vi "Configure Chan Group.vi"(8 "error in (no error)":errorcluster, 11 "Cfg Grandmaster in":refnum<class "Cfg Grandmaster.lvclass">) -> (0 "error out":errorcluster, 3 "Cfg Grandmaster out":refnum<class "Cfg Grandmaster.lvclass">)   [LabVIEW 2018, in "Configuration Grandmaster.lvlib" / "Cfg Grandmaster.lvclass"]
uses:
  Cfg Grandmaster.lvclass
  Cfg Grandmaster.lvclass/Cfg Grandmaster.ctl
  Class Chassis BOM/Chassis BOM.lvclass/Chassis BOM.ctl
  Class Chassis BOM/Read Chassis Alias.vi
  Class Chassis Cfg/ChassisCfg.lvclass
  Class Chassis BOM/Chassis BOM.lvclass
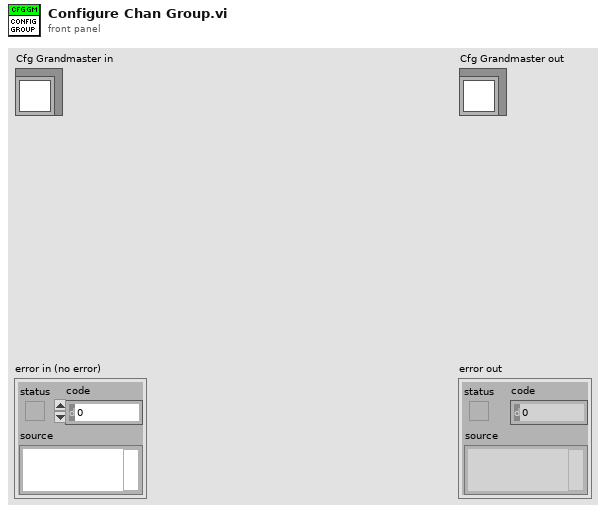
[diagram p1: front panel]
types:
  T1 = typedef "DAQMan Mode.ctl" = enum16{"Cfg", "Run", "Shutting Down"}
  T2 = typedef "ge_Cfg wChassis.ctl" = cluster{"Chassis BOM":refnum<class "Chassis BOM.lvclass">, "Chassis Cfg":refnum<class "ChassisCfg.lvclass">, "Chassis Tasks":refnum<class "Chassis Tasks.lvclass">, "HW Error":bool, "Unsvd Chgs?":bool}
  T3 = typedef "Selected Group.ctl" = cluster{"ChanGroup":i32, "Rate Class":T4}
  T4 = typedef "TE_Designator.ctl" = enum16{"High Speed", "Low Speed"}
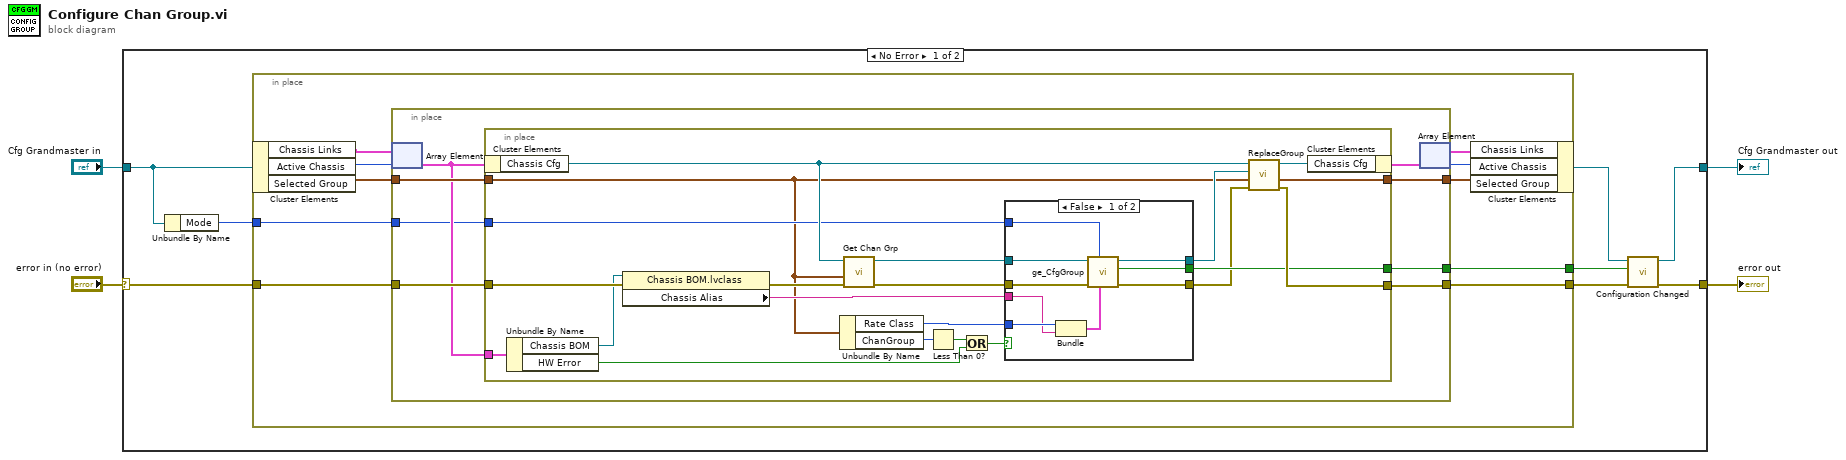
[diagram p0: block diagram]
diagram:
  n1 = case shown="No Error" "error in (no error)" {
    selector: "error in (no error)" -> [w12 w65]
    tunnel: [w8 w65] -> w3
    tunnel: [w5 w64] -> w1
    tunnel: "Cfg Grandmaster in" -> [w11 w64]
    frame No Error {
      n2 = Unbundle By Name(w11) -> ("Mode"=w10:T1)
      n3 = in-place {
        in-place-border: w12 -> [w20]
        in-place-border: [w16] -> w9
        in-place-border: w10 -> [w15]
        in-place-border: [w13] -> w7
        n4 = in-place-cluster #1(w11) -> ("Chassis Links"=w22:T2[], "Active Chassis"=w21:i32, "Selected Group"=w17:T3)
        n5 = in-place {
          in-place-border: [w30] -> w16
          in-place-border: [w29] -> w13
          in-place-border: w20 -> [w28]
          in-place-border: w17 -> [w27]
          in-place-border: w15 -> [w24]
          in-place-border: [w23] -> w14
          n6 = in-place-array #2(w22, w21) -> (w26:T2)
          n7 = in-place {
            in-place-border: [w51] -> w30
            in-place-border: [w50] -> w29
            in-place-border: w28 -> [w38]
            in-place-border: w27 -> [w32]
            in-place-border: w26 -> [w42]
            in-place-border: w24 -> [w34]
            in-place-border: [w31] -> w23
            n8 = in-place-cluster #3(w26) -> ("Chassis Cfg"=w39:refnum<class "ChassisCfg.lvclass">)
            n9 = Unbundle By Name(w42) -> ("Chassis BOM"=w36:refnum<class "Chassis BOM.lvclass">, "HW Error"=w41:bool)
            n10 = property class="Chassis BOM.lvclass"(reference=w36, error in=w38) -> (error out=w37:errorcluster, "Chassis Alias"=w35:string)  [unwired: 1 out]
            n11 = Unbundle By Name(w32) -> ("Rate Class"=w45:T4, "ChanGroup"=w49:i32)
            n12 = call "Get Chan Grp.vi"("error in (no error)"=w37, "Selected Grp"=w32, "Chassis Cfg"=w39) -> ("error out"=w44:errorcluster, "Chan Group"=w48:refnum<class "ChanGrp.lvclass">)  [unwired: 7 in]
            n13 = Less Than 0?(x=w49) -> (x < 0?=w47:bool)
            n14 = Or(x=w47, y=w41) -> (x .or. y?=w46:bool)
            n15 = case shown="False" w46 {
              selector: w46 -> [_ w61]
              tunnel: w44 -> [w59 w63]
              tunnel: [w60 w63] -> w43
              tunnel: w48 -> [w58 w62]
              tunnel: [w57 w62] -> w33
              tunnel: [w52 w61] -> w50
              tunnel: w34 -> [w56 _]
              tunnel: w45 -> [w55 _]
              tunnel: w35 -> [w54 _]
              frame False {
                n16 = Bundle("Rate Class"=w55, "Chassis Alias"=w54) -> (w53:cluster{"Rate Class":T4, "Chassis Alias":string})  [unwired: 1 in]
                n17 = call "ge_CfgGroup.vi"("Group Specific Info"=w53, "Mode"=w56, "error in"=w59, "ChanGrp.lvclass"=w58) -> ("error out"=w60:errorcluster, "Canceled?"=w52:bool, "ChanGrp.lvclass"=w57:refnum<class "ChanGrp.lvclass">)  [unwired: 5 in]
              }
              frame True {
              }
            }
            n18 = call "ReplaceGroup.vi"("error in (no error)"=w43, "Selected Grp"=w32, "Group Info"=w33, "Chassis Cfg"=w39) -> ("error out"=w51:errorcluster, "Selected Grp"=w31:T3, "Chassis Cfg"=w40:refnum<class "ChassisCfg.lvclass">)  [unwired: 5 in]
            n19 = in-place-cluster #3("Chassis Cfg"=w40) -> (w25:T2)
          }
          n20 = in-place-array #2(w25) -> (w19:T2[], w18:i32)
        }
        n21 = in-place-cluster #1("Chassis Links"=w19, "Active Chassis"=w18, "Selected Group"=w14) -> (w6:refnum<class "Cfg Grandmaster.lvclass">)
      }
      n22 = call "Configuration Changed.vi"("error in (no error)"=w9, "Canceled? (F)"=w7, "Cfg Grandmaster in"=w6) -> ("error out"=w8:errorcluster, "Cfg Grandmaster out"=w5:refnum<class "Cfg Grandmaster.lvclass">)  [unwired: 7 in]
    }
    frame Error {
    }
  }
  "error out" <- w3
  "Cfg Grandmaster out" <- w1
